vi "DP-Read Data.vi"(0 "Path":path, 11 "error in":errorcluster) -> (4 "Data matrix":dbl[][](array[numeric]), 8 "F2 array":dbl[](array[numeric]), 10 "L2 array":dbl[](array[numeric]), 15 "error out":errorcluster)   [LabVIEW 2020]
uses:
  <vilib>/Analysis/polynomials.llb/Unique Numbers and Multiplicity (DBL).vi
  <vilib>/Analysis/NI_AALPro.lvlib
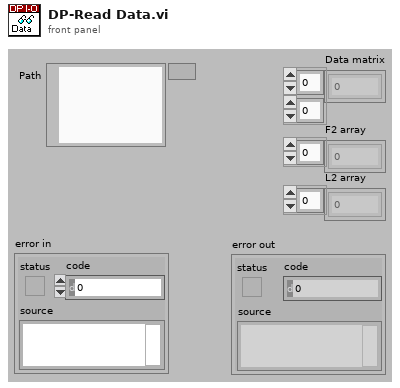
[diagram p1: front panel]
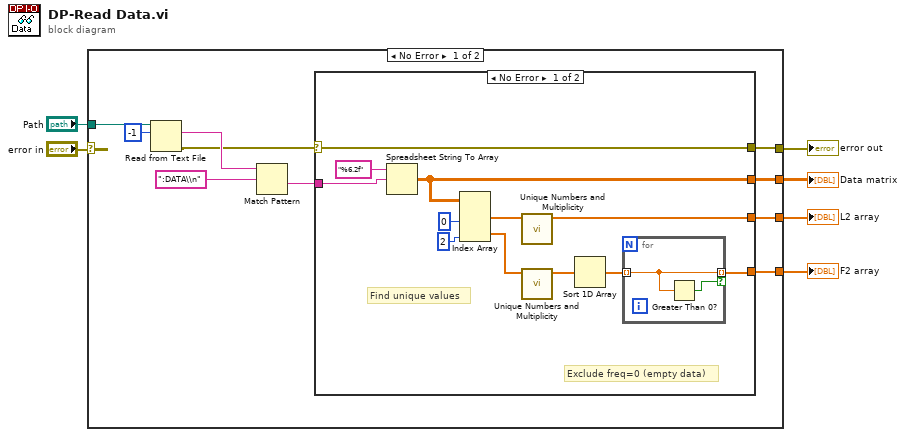
[diagram p0: block diagram]
diagram:
  n1 = case shown="No Error" "error in" {
    tunnel: "Path" -> [w9 _]
    tunnel: [w16 _] -> w4
    tunnel: [w15 _] -> w3
    tunnel: [w14 _] -> w2
    tunnel: [w13 _] -> w1
    frame No Error {
      n2 = Read from Text File(file (use dialog)=w9, count=-1) -> (text=w12:string, error out=w7:errorcluster)  [unwired: 2 in, 2 out]
      n3 = Match Pattern(string=w12, regular expression=":DATA\\n") -> (after substring=w8:string)  [unwired: 1 in, 3 out]
      n4 = case shown="No Error" w7 {
        selector: w7 -> [w26 w31]
        tunnel: w8 -> [w28 _]
        tunnel: [w22 _] -> w16
        tunnel: [w26 w31] -> w15
        tunnel: [w23 _] -> w14
        tunnel: [w17 _] -> w13
        frame No Error {
          # "Exclude freq=0 (empty data)"
          # "Find unique values"
          n5 = Spreadsheet String To Array(format string="%6.2f", spreadsheet string=w28) -> (array=w22:dbl[][])  [unwired: 2 in]
          n6 = Index Array(array=w22, index (col) #1=0 ("disabled index (col)"), index (col) #2=2 ("disabled index (col)")) -> (element #1=w24:dbl[], element #2=w19:dbl[])  [unwired: 2 in]
          n7 = call-poly <vilib>:"Unique Numbers and Multiplicity.vi"("Numbers"=w24) -> ("Unique Numbers"=w23:dbl[])  [unwired: 8 in, 2 out]
          n8 = call-poly <vilib>:"Unique Numbers and Multiplicity.vi"("Numbers"=w19) -> ("Unique Numbers"=w21:dbl[])  [unwired: 8 in, 2 out]
          n9 = Sort 1D Array(array=w21) -> (sorted array=w18:dbl[])
          n10 = for {
            tunnel: w18 -> [w29] mode=indexing
            tunnel: [w29] -> w17 mode=indexing if=w30
            n11 = Greater Than 0?(x=w29) -> (x > 0?=w30:bool)
          }
        }
        frame Error {
        }
      }
    }
    frame Error {
    }
  }
  "error out" <- w3
  "Data matrix" <- w4
  "F2 array" <- w1
  "L2 array" <- w2
